vi "test_resist_old.vi"() -> ()   [LabVIEW 2015]
uses:
  global_qaqc.vi
panel:
  out "File Path Out":path
  in  "?":bool
  out "Last value (MOhm)":dbl
  out "Name of PCB":string
  out "Boolean 16":bool
  out "Boolean 15":bool
  out "Boolean 14":bool
  out "Boolean 13":bool
  out "Boolean 12":bool
  out "Boolean 11":bool
  out "Boolean 10":bool
  out "Boolean 9":bool
  out "Boolean 8":bool
  out "Boolean 7":bool
  out "Boolean 6":bool
  out "Boolean 5":bool
  out "Boolean 4":bool
  out "Boolean 3":bool
  out "Boolean 2":bool
  out "Boolean":bool
  in  "Open Database":bool
  in  "Close VI":bool
  in  "?":bool
  # "1) Setup the measure and then click \"Acquire\". If you want to take again the last measure, click \"Redo last\" and then \"Acquire\""
  # "Yellow: Done"
  # "Green: OK"
  # "Yellow: Done"
  # "Green: OK"
  # "Circular small LED \n\nGREY --> Measure NOT DONE\nYELLOW --> Measure DONE\n\n\nElliptic big LED\n\nRED --> Value not taken OR out of range\nGREEN --> Value in range"
  # "2) Once measure is finished, open the database and upload the file"
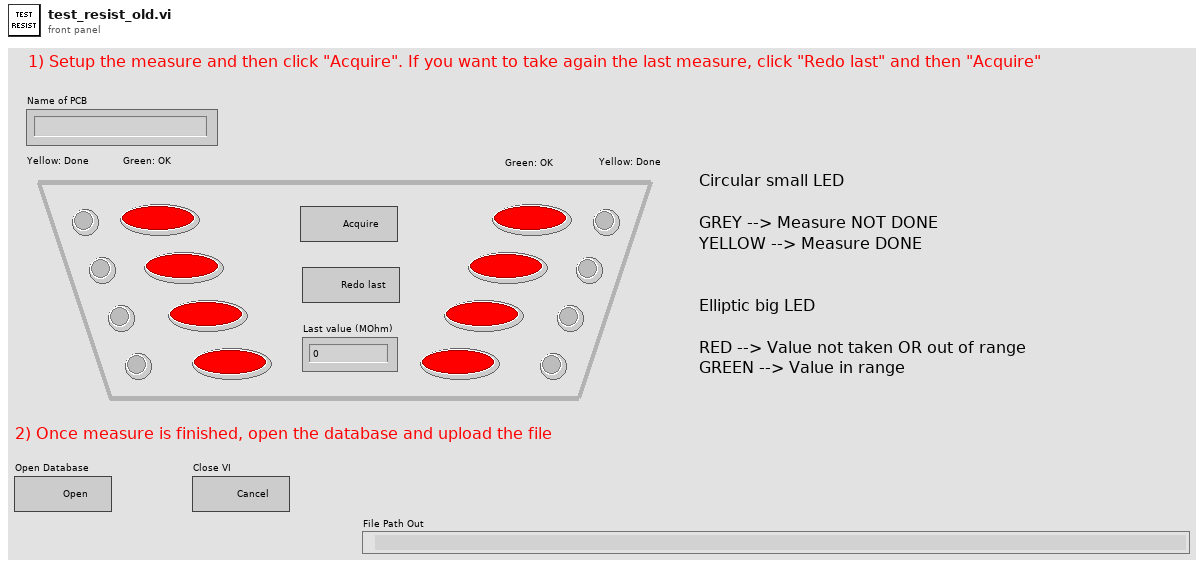
[diagram p1: front panel]
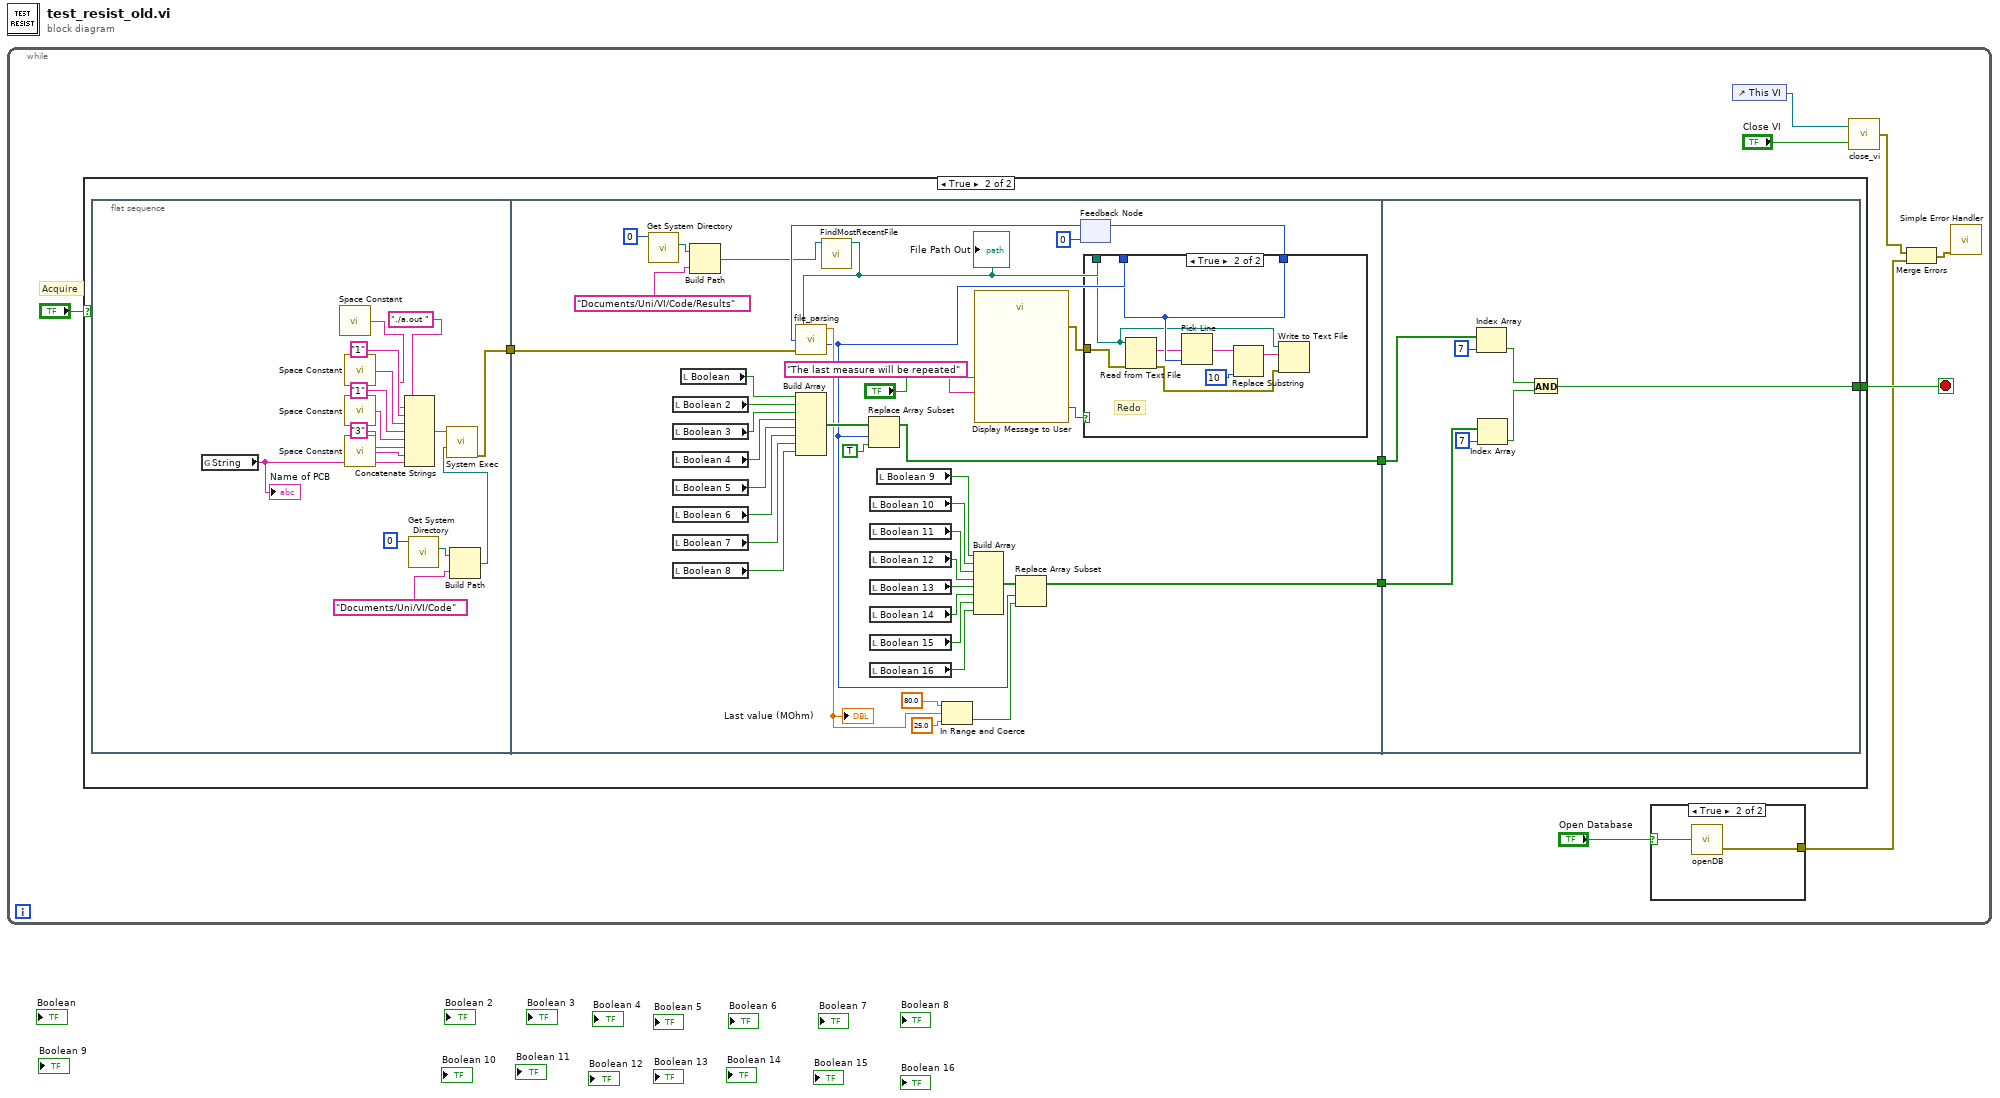
[diagram p0: block diagram]
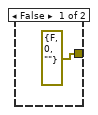
[diagram p2: hidden frame]
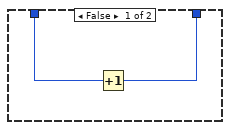
[diagram p4: hidden frame]
diagram:
  n1 = while {
    stop <- w4 stop-if-true
    # "Acquire"
    n2 = case shown="True" "?" {
      selector: "?" -> [w12 _]
      tunnel: [w12 w14] -> w4
      frame False {
      }
      frame True {
        n3 = flat-sequence {
          tunnel: [w24] -> w13
          tunnel: [w44] -> w16
          tunnel: [w43] -> w15
          tunnel: w13 -> [w70]
          tunnel: w16 -> [w85]
          tunnel: w15 -> [w84]
          tunnel: [w81] -> w14
          frame #0 {
            n4 = global read "global_qaqc.vi" "String"() -> (w31:string)
            "Name of PCB" <- w31
            n5 = call <vilib>:"Space Constant.vi"() -> ("String"=w23:string)
            n6 = call <vilib>:"Space Constant.vi"() -> ("String"=w25:string)
            n7 = call <vilib>:"Space Constant.vi"() -> ("String"=w26:string)
            n8 = call <vilib>:"Space Constant.vi"() -> ("String"=w30:string)
            n9 = Concatenate Strings("./a.out " ("String"), w23, "1", w25, "1", w26, "3", w30, w31) -> (w17:string)
            n10 = call <vilib>:"Get System Directory.vi"("system directory type"=0) -> ("system directory"=w20:path)  [unwired: 10 in]
            n11 = Build Path(base path=w20, name or relative path="Documents/Uni/VI/Code") -> (appended path=w18:path)
            n12 = call <vilib>:"System Exec.vi"("working directory"=w18, "command line"=w17) -> ("error out"=w24:errorcluster)  [unwired: 6 in, 3 out]
          }
          frame #1 {
            n13 = call <vilib>:"Get System Directory.vi"("system directory type"=0) -> ("system directory"=w35:path)  [unwired: 10 in]
            n14 = local read "Boolean 2"() -> (w63:bool)
            n15 = local read "Boolean 3"() -> (w64:bool)
            n16 = local read "Boolean 4"() -> (w65:bool)
            n17 = local read "Boolean 5"() -> (w66:bool)
            n18 = local read "Boolean 6"() -> (w67:bool)
            n19 = local read "Boolean 7"() -> (w68:bool)
            n20 = local read "Boolean 8"() -> (w69:bool)
            n21 = local read "Boolean"() -> (w62:bool)
            n22 = Build Path(base path=w35, name or relative path="Documents/Uni/VI/Code/Results") -> (appended path=w33:path)
            n23 = Build Array(w62, w63, w64, w65, w66, w67, w68, w69) -> (w59:bool[])
            n24 = call "FindMostRecentFile.vi"("Folder Path In"=w33) -> ("File Path Out"=w32:path)  [unwired: 9 in, 1 out]
            "File Path Out" <- w32
            n25 = local read "Boolean 10"() -> (w54:bool)
            n26 = local read "Boolean 11"() -> (w53:bool)
            n27 = local read "Boolean 12"() -> (w52:bool)
            n28 = local read "Boolean 13"() -> (w51:bool)
            n29 = local read "Boolean 14"() -> (w50:bool)
            n30 = local read "Boolean 15"() -> (w49:bool)
            n31 = local read "Boolean 16"() -> (w48:bool)
            n32 = local read "Boolean 9"() -> (w55:bool)
            n33 = Build Array(w55, w54, w53, w52, w51, w50, w49, w48) -> (w47:bool[])
            n34 = call "Display Message to User"("Enable"="?", "Message"="The last measure will be repeated") -> ("error out"=w37:errorcluster, "OK"=w42:bool)  [unwired: 8 in]
            n35 = feedback #1(0) -> (w60:i32)
            n36 = call "file_parsing.vi"("File Path Control"=w32, "line index"=w60, "error in"=w70) -> ("Waveform Chart"=w45:dbl, "index output"=w39:i32)  [unwired: 2 out]
            "Last value (MOhm)" <- w45
            n37 = Replace Array Subset(array=w59, new element=TRUE ("new element/subarray"), index=w39) -> (w44:bool[])
            n38 = In Range and Coerce(upper limit=80.0, x=w45, lower limit=25.0) -> (In Range?=w46:bool)  [unwired: 1 out]
            n39 = Replace Array Subset(array=w47, new element=w46, index=w39) -> (w43:bool[])
            n40 = case shown="True" w42 {
              tunnel: w39 -> [w72 w80]
              tunnel: [w71 w80] -> w38
              tunnel: w32 -> [_ w77]
              tunnel: w37 -> [_ w75]
              frame False {
                n41 = Increment(x=w72) -> (x+1=w71:i32)
              }
              frame True {
                # "Redo"
                n42 = Read from Text File(file (use dialog)=w77, error in=w75) -> (text=w73:string, error out=w74:errorcluster)  [unwired: 2 in, 2 out]
                n43 = Pick Line(multi-line string=w73, line index=w80) -> (output string=w79:string)  [unwired: 1 in]
                n44 = Replace Substring(2:10 ("length (len. of substring)"), 5:w79) -> (1:w78:string)  [unwired: 2 in, 1 out]
                n45 = Write to Text File(file (use dialog)=w77, text=w78, error in=w74) -> ()  [unwired: 1 in, 3 out]
              }
            }
            n46 = feedback-in #1(w38) -> ()
          }
          frame #2 {
            n47 = Index Array(array=w85, index=7) -> (element=w83:bool)
            n48 = Index Array(array=w84, index=7) -> (element=w82:bool)
            n49 = And(x=w83, y=w82) -> (x .and. y?=w81:bool)
          }
        }
      }
    }
    n50 = case shown="True" "Open Database" {
      selector: "Open Database" -> [_ w11]
      tunnel: [errorcluster {"status"=FALSE, "code"=0, "source"=""} ("error out") w10] -> w3
      frame False {
      }
      frame True {
        n51 = call "openDB.vi"("Open Button"=w11) -> ("error out"=w10:errorcluster)  [unwired: 1 out]
      }
    }
    n52 = control-ref of="This VI"() -> (w6:refnum<vi>)
    n53 = call "close_vi.vi"("Process Stop Button"="Close VI", "reference"=w6) -> ("error out"=w1:errorcluster)
    n54 = Merge Errors(w1, w3) -> (w2:errorcluster)
    n55 = call <vilib>:"Simple Error Handler.vi"("error in (no error)"=w2) -> ()  [unwired: 4 in, 5 out]
  }
